vi "1A_BFG Ramp Data.vi"(7 "array":dbl[][](array[numeric])) -> (8 "Threshold Values":u16[](array[numeric]))   [LabVIEW 2010]
panel:
  # "•\tBattery 75% Voltage Threshold, No Load: 3.950V\n•\tBattery 75% Voltage Threshold, Stimulation On: 3.925V\n•\tBattery 50% Voltage Threshold, No Load: 3.850V\n•\tBattery 50% Voltage Threshold, Stimulation On: 3.825V\n•\tBattery 25% Voltage Threshold, No Load: 3.780V\n•\tBattery 25% Voltage Threshold, Stimulation On: 3.755V\n•\tBattery Warning Voltage Threshold, No Load: 3.740V\n•\tBattery Warning Voltage Threshold, Stimulation On: 3.715V\n•\tBattery Critical Voltage Threshold, No Load: 3.720V\n•\tBattery Critical Voltage Threshold, Stimulation On: 3.695V\n•\tMinimum Safe Stimulating Voltage, No Load: 3.700V\n•\tMinimum Safe Stimulation Voltage, Stimulation On: 3.675V\n•\tBattery Cut-off Voltage Threshold:  2.850V"
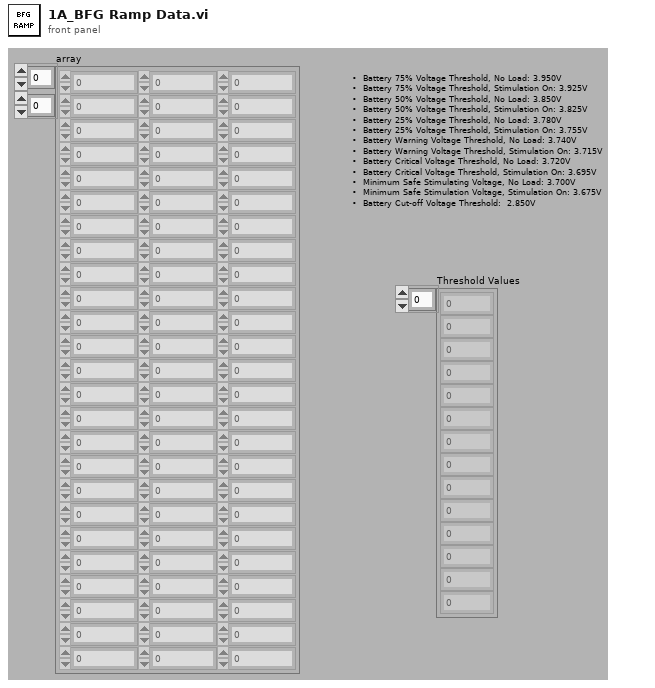
[diagram p1: front panel]
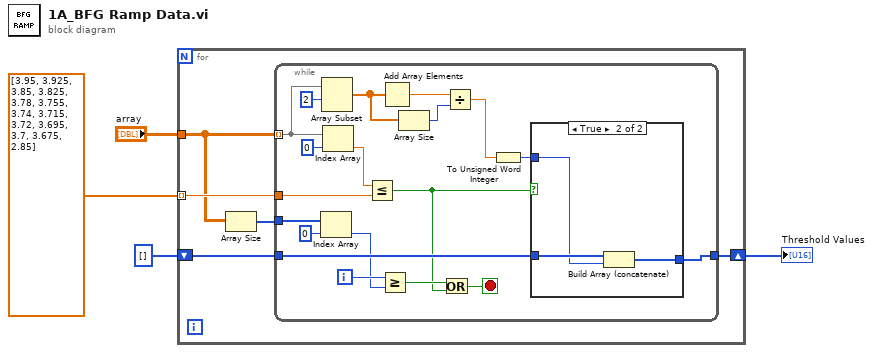
[diagram p0: block diagram]
diagram:
  n1 = for {
    tunnel: dbl[] [3.95, 3.925, 3.85, 3.825, 3.78, 3.755, 3.74, 3.715, 3.72, 3.695, 3.7, 3.675, 2.85] -> [w9] mode=indexing
    shift-right: [w7] -> w3
    shift-left: u16[] [] -> [w8]
    tunnel: "array" -> [w5]
    n2 = Array Size(array=w5) -> (size(s)=w6:i32[])
    n3 = while {
      tunnel: w5 -> [w14] mode=indexing
      tunnel: w9 -> [w25]
      tunnel: w8 -> [w24]
      tunnel: [w23] -> w7
      tunnel: w6 -> [w22]
      i -> [w17]
      stop <- w18 stop-if-true
      n4 = Index Array(array=w22, index=0) -> (element=w16:i32)
      n5 = Array Subset(array=w14, index=2) -> (w13:dbl[])  [unwired: 1 in]
      n6 = Index Array(array=w14, index=0) -> (element=w27:dbl)
      n7 = Less Or Equal?(x=w27, y=w25) -> (x <= y?=w19:bool)
      n8 = Greater Or Equal?(x=w17, y=w16) -> (x >= y?=w20:bool)
      n9 = Add Array Elements(numeric array=w13) -> (sum=w11:dbl)
      n10 = Array Size(array=w13) -> (size(s)=w12:i32)
      n11 = Or(x=w20, y=w19) -> (x .or. y?=w18:bool)
      n12 = Divide(x=w11, y=w12) -> (x/y=w10:dbl)
      n13 = To Unsigned Word Integer(number=w10) -> (unsigned 16bit integer=w26:u16)
      n14 = case shown="True" w19 {
        tunnel: w26 -> [_ w30]
        tunnel: w24 -> [w29 w32]
        tunnel: [w29 w31] -> w23
        frame False {
        }
        frame True {
          n15 = Build Array (concatenate)(w32, w30) -> (w31:u16[])
        }
      }
    }
  }
  "Threshold Values" <- w3
